vi "Actor Core.vi"(8 "error in":errorcluster, 11 "State in":refnum<class "Drive Train.lvclass">) -> (0 "error out":errorcluster, 3 "Actor out":refnum<class "Actor.lvclass">)   [LabVIEW 2013, in "Logical Systems.lvlib" / "Drive Train.lvlib" / "Drive Train.lvclass"]
doc: "(<B>Filename</B>: Actor Framework.lvlib:Actor.lvclass:Actor Core.vi)\n\nThis override invokes Entry.vi on the initial state, prior to calling the parent Actor Core. Adding this behavior to Actor Core (instead of an override of Pre Launch Init.vi) allows the initial state to launch a nested actor as part of its entry behavior.\n\nReceives messages to the actor, reacts to them, and initiates any error handling that may shut the actor down.\n\nDescendant classes may override this VI to append parallel tasks for the actor to complete while it handles messages. Overrides use the Call Parent Method node."
uses:
  Drive Train.lvclass
  <vilib>/ActorFramework/Actor/Actor.lvclass
  Drive Train Status.ctl
  Drive Train.lvclass/Drive Train.ctl
  Robot Actors/System Actor/System Actor Class/System Actor.lvclass
panel:
  in  "Drive Train Status":T1 {"Right Power Setpoint" min=-1.0 max=1.0 step=0.1 scale=-1.0..1.0; "Left Power Setpoint" min=-1.0 max=1.0 step=0.1 scale=-1.0..1.0; "Right Power" min=-1.0 max=1.0 step=0.1 scale=-1.0..1.0; "Left Power" min=-1.0 max=1.0 step=0.1 scale=-1.0..1.0}
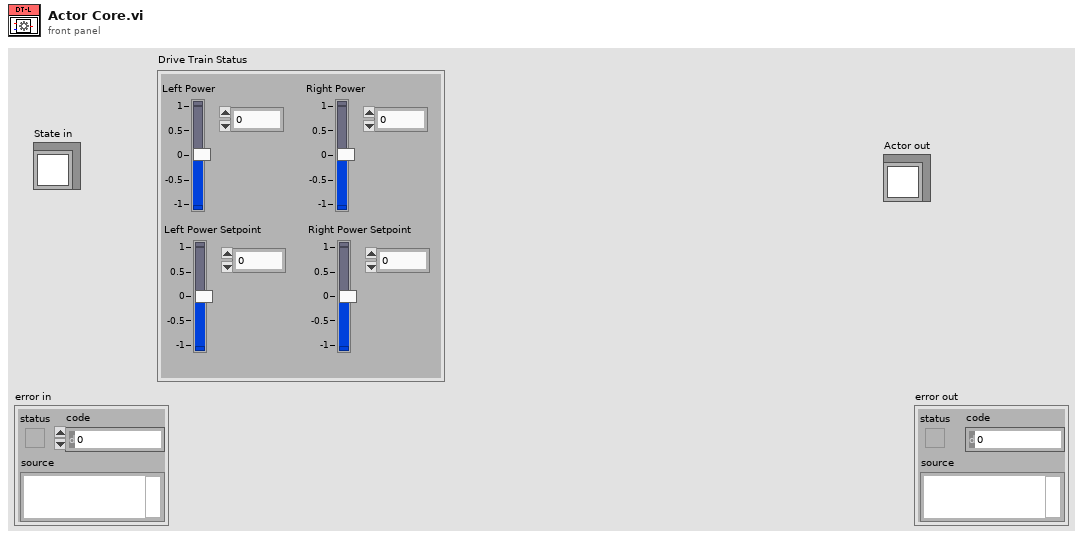
[diagram p1: front panel]
types:
  T1 = typedef "Logical Systems.lvlib/Drive Train.lvlib/Drive Train.lvclass/Drive Train Status.ctl" = cluster{"Left Power":dbl, "Right Power":dbl, "Left Power Setpoint":dbl, "Right Power Setpoint":dbl}
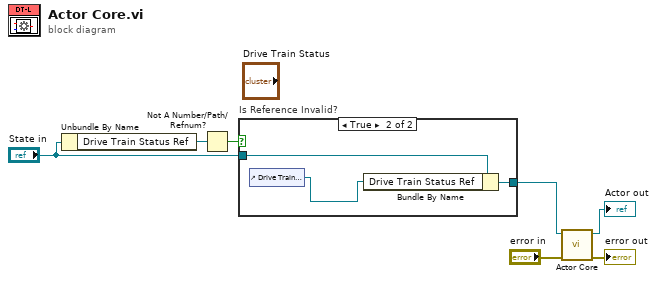
[diagram p0: block diagram]
diagram:
  n1 = Unbundle By Name("State in") -> ("Drive Train Status Ref"=w2:refnum<vi>)
  n2 = Not A Number/Path/Refnum?(number/path/refnum=w2) -> (NaN/Path/Refnum?=w1:bool)
  n3 = case "Is Reference Invalid?" shown="True" w1 {
    tunnel: [w8 w11] -> w4
    tunnel: "State in" -> [w8 w10]
    frame False {
    }
    frame True {
      n4 = control-ref of="Drive Train Status"() -> (w9:refnum<vi>)
      n5 = Bundle By Name(cluster=w10, "Drive Train Status Ref"=w9) -> (w11:refnum<class "Drive Train.lvclass">)
    }
  }
  n6 = call-parent "Actor Core.vi"("error in"="error in", "State in"=w4) -> ("error out"=→"error out":errorcluster, "Actor out"=→"Actor out":refnum<class "Actor.lvclass">)  [unwired: 8 in]
